vi "Destroy.vi"(0 "reference in":refnum<class "AnotherClass.lvclass">, 5 "error in (no error)":errorcluster) -> (14 "reference out":refnum<class "AnotherClass.lvclass">, 19 "error out":errorcluster)   [LabVIEW 2020, in "AnotherClass.lvclass"]
uses:
  <vilib>/addons/GOOPUtility/_Demo/GOOPUtil_Demo/AnotherClass_class/AnotherClass.lvclass
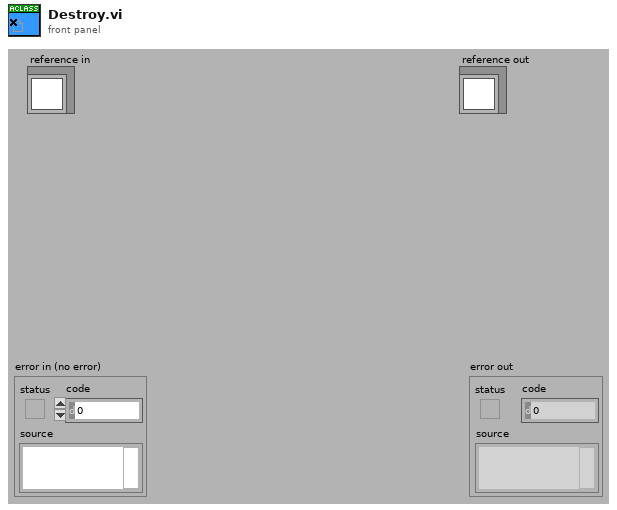
[diagram p1: front panel]
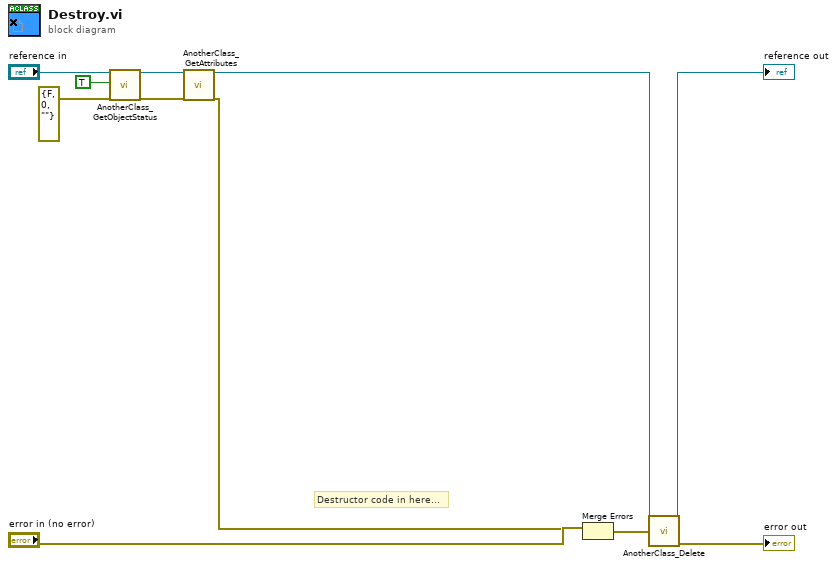
[diagram p0: block diagram]
diagram:
  # "Destructor code in here..."
  n1 = call <vilib>:"AnotherClass_GetObjectStatus.vi"("reference in"="reference in", "Simple Info"=TRUE, "error in (no error)"=errorcluster {"status"=FALSE, "code"=0, "source"=""}) -> ("reference out"=w5:refnum<class "AnotherClass.lvclass">, "error out"=w2:errorcluster)  [unwired: 6 in, 9 out]
  n2 = call <vilib>:"AnotherClass_GetAttributes.vi"("reference in"=w5, "error in (no error)"=w2) -> ("reference out"=w9:refnum<class "AnotherClass.lvclass">, "error out"=w7:errorcluster)  [unwired: 14 in, 2 out]
  n3 = Merge Errors("error in (no error)", w7) -> (w8:errorcluster)
  n4 = call <vilib>:"AnotherClass_Delete.vi"("reference in"=w9, "error in (no error)"=w8) -> ("reference out"=→"reference out":refnum<class "AnotherClass.lvclass">, "error out"=→"error out":errorcluster)  [unwired: 15 in, 1 out]
